vi "Check Pattern Name.vi"(8 "error in (no error)":errorcluster, 10 "Pattern Name":string, 11 "File Parser Interface in":refnum<class "File Parser Interface.lvclass">) -> (0 "error out":errorcluster, 3 "File Parser Interface out":refnum<class "File Parser Interface.lvclass">)   [LabVIEW 2018, in "File Parser Interface.lvlib" / "File Parser Interface.lvclass"]
uses:
  File Parser Interface.lvclass
  File Parser Interface.lvclass/File Parser Interface.ctl
  Read File Path.vi
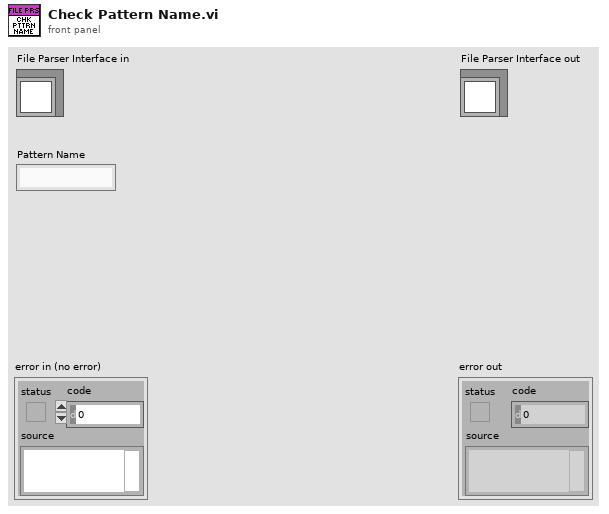
[diagram p1: front panel]
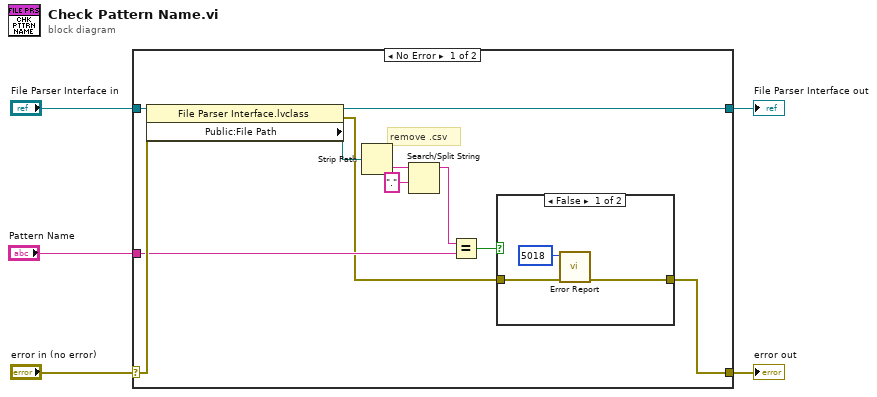
[diagram p0: block diagram]
diagram:
  n1 = case shown="No Error" "error in (no error)" {
    selector: "error in (no error)" -> [w15 w22]
    tunnel: [w6 w22] -> w4
    tunnel: [w8 w21] -> w2
    tunnel: "File Parser Interface in" -> [w16 w21]
    tunnel: "Pattern Name" -> [w10 _]
    frame No Error {
      # "remove .csv"
      n2 = property class="File Parser Interface.lvclass"(reference=w16, error in=w15) -> (reference out=w8:refnum<class "File Parser Interface.lvclass">, error out=w7:errorcluster, "Public:File Path"=w14:path)
      n3 = Strip Path(path=w14) -> (name=w13:string)  [unwired: 1 out]
      n4 = Search/Split String(string=w13, search string/char (-)=".") -> (substring before match=w11:string)  [unwired: 1 in, 2 out]
      n5 = Equal?(x=w11, y=w10) -> (x = y?=w9:bool)
      n6 = case shown="False" w9 {
        tunnel: w7 -> [w19 w20]
        tunnel: [w17 w20] -> w6
        frame False {
          n7 = call "Error Report.vi"("error in (no error)"=w19, "Error Code"=i16 5018) -> ("error out"=w17:errorcluster)  [unwired: 9 in]
        }
        frame True {
        }
      }
    }
    frame Error {
    }
  }
  "error out" <- w4
  "File Parser Interface out" <- w2
